vi "log_file_to_display_data.vi"(11 "Master Log":string[][](table)) -> (3 "Formatted table":string[][](table))   [LabVIEW 2016]
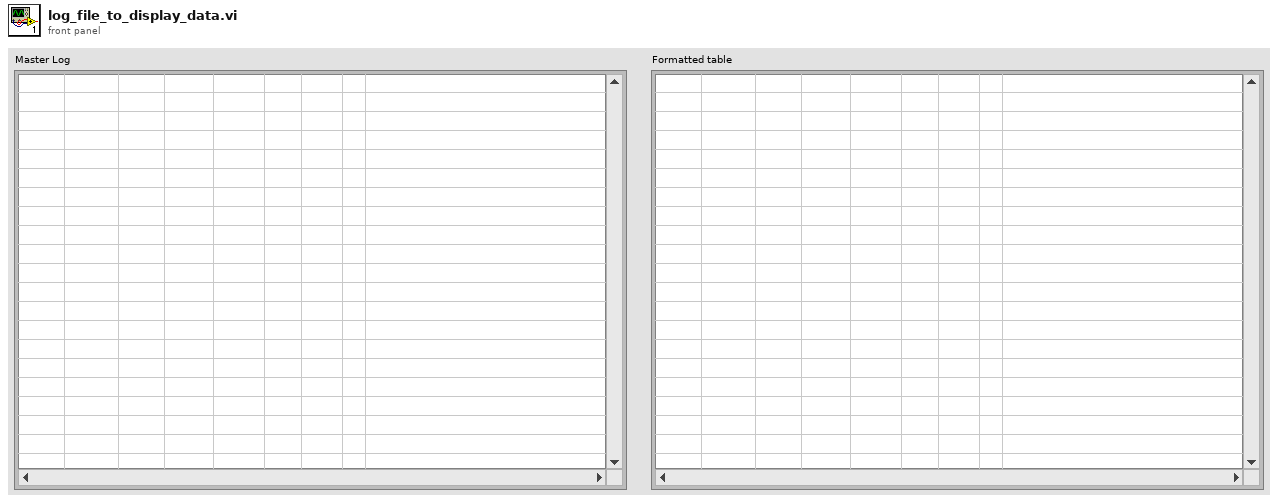
[diagram p1: front panel]
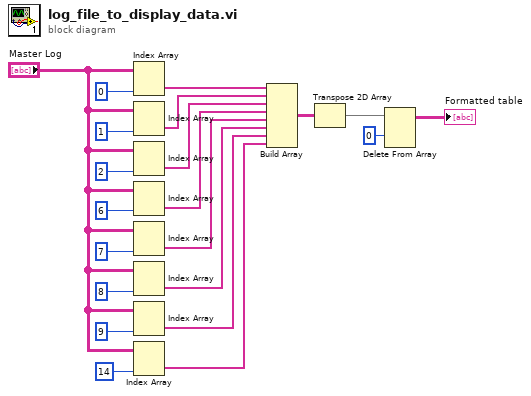
[diagram p0: block diagram]
diagram:
  n1 = Index Array(array="Master Log", index (col)=0) -> (element=w12:string[])  [unwired: 1 in]
  n2 = Index Array(array="Master Log", index (col)=1) -> (element=w11:string[])  [unwired: 1 in]
  n3 = Index Array(array="Master Log", index (col)=2) -> (element=w10:string[])  [unwired: 1 in]
  n4 = Index Array(array="Master Log", index (col)=6) -> (element=w9:string[])  [unwired: 1 in]
  n5 = Index Array(array="Master Log", index (col)=7) -> (element=w8:string[])  [unwired: 1 in]
  n6 = Index Array(array="Master Log", index (col)=8) -> (element=w7:string[])  [unwired: 1 in]
  n7 = Index Array(array="Master Log", index (col)=9) -> (element=w6:string[])  [unwired: 1 in]
  n8 = Index Array(array="Master Log", index (col)=14) -> (element=w5:string[])  [unwired: 1 in]
  n9 = Build Array(w12, w11, w10, w9, w8, w7, w6, w5) -> (w4:string[][])
  n10 = Transpose 2D Array(2D array=w4) -> (transposed array=w3:string[][])
  n11 = Delete From Array(array=w3, index (row)=0) -> (array with subset deleted=→"Formatted table":string[][])  [unwired: 2 in, 1 out]
